vi "SimHallSensor.vi"() -> ()   [LabVIEW 2014]
doc: "Use this template to build a user interface event handler design pattern. Use this pattern for dialog boxes and other user interfaces. You also can create and execute user-defined events that the VI can handle the same way as user interface events."
uses:
  subVIs/SimHallSensor.ctl
  <vilib>/Utility/error.llb/DialogType.ctl
  <vilib>/DAQmx/create/channels.llb/DAQmx Create Channel (AO-Voltage-Basic).vi
  <vilib>/DAQmx/configure/timing.llb/DAQmx Timing (Sample Clock).vi
  <resource>/objmgr/daqmx.rc
panel:
  in  "Pulse Params":T1={"Amplitude"=5.0, "Duty Cycle"=0.1, "Shape"=enum."Square"}
  in  "Speed (RPM)":dbl(knob) scale=300.0..20000.0 scale format="%#_3p"
  in  "Engage":bool
  in  "DAQ Parameters":T2={"physical channels"="", "maximum value"=5.0, "minimum value"=-5.0, "rate"=100000.0, "buffer len"=1.0} {"buffer len" format="%0.2f"; "rate" format="%.1p"; "minimum value" format="%0.2f"; "maximum value" format="%0.2f"}
  out "Waveform Graph":waveform(dbl)(graph)
  in  "quit":bool
  # "V"
  # "V"
  # "Hz"
  # "s"
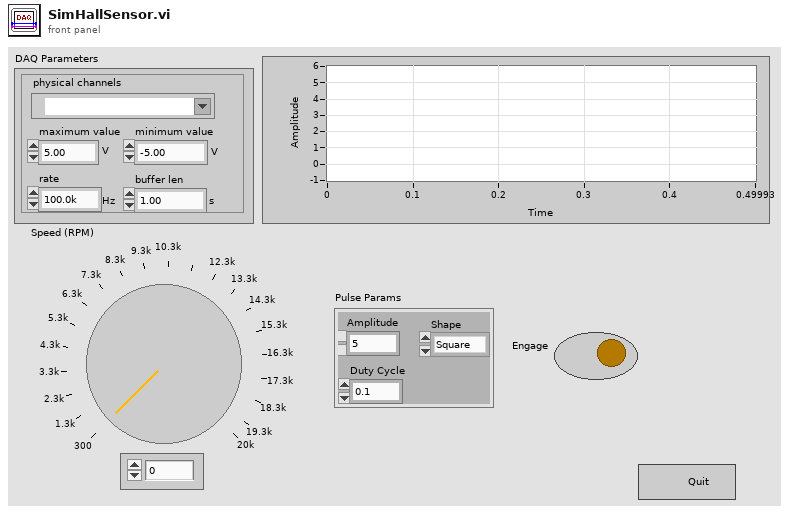
[diagram p1: front panel]
types:
  T1 = cluster{"Amplitude":dbl, "Duty Cycle":dbl, "Shape":enum16{"Square", "Cosine"}}
  T2 = cluster{"physical channels":tag, "maximum value":dbl, "minimum value":dbl, "rate":dbl, "buffer len":dbl}
  T3 = typedef "SimHallSensor.ctl" = enum16{"Init", "Idle", "CheckError", "Finalize", "ConfigDAQ", "StartDAQ", "Monitor", "StopDAQ", "ClearDAQ"}
  T4 = typedef "DialogType.ctl" = u16
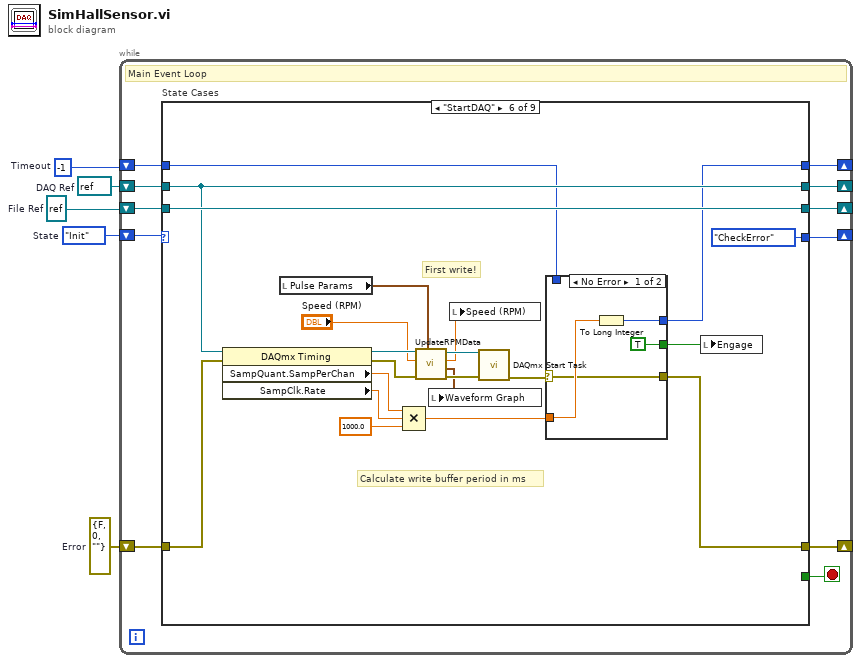
[diagram p0: block diagram]
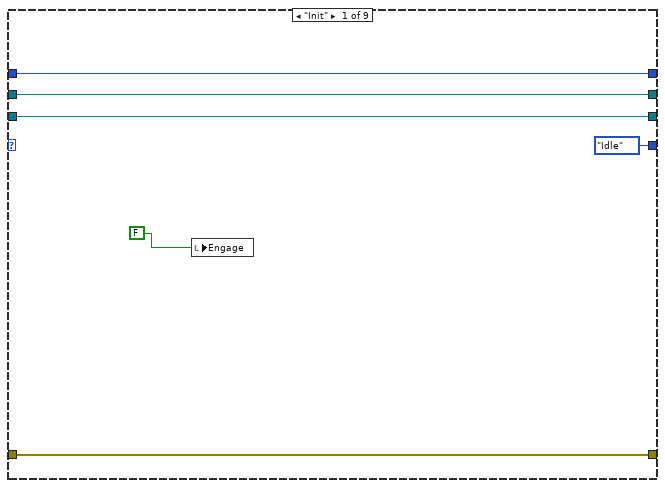
[diagram p2: hidden frame]
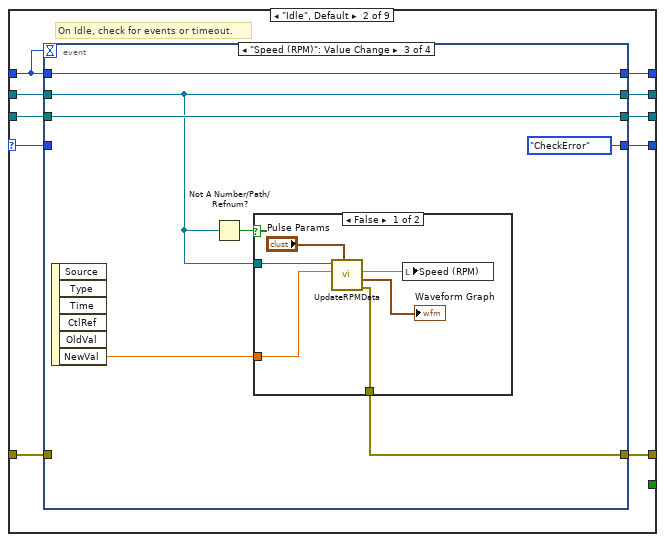
[diagram p3: hidden frame]
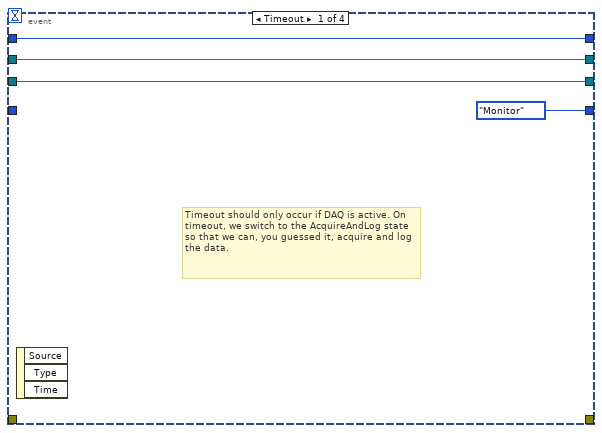
[diagram p4: hidden frame]
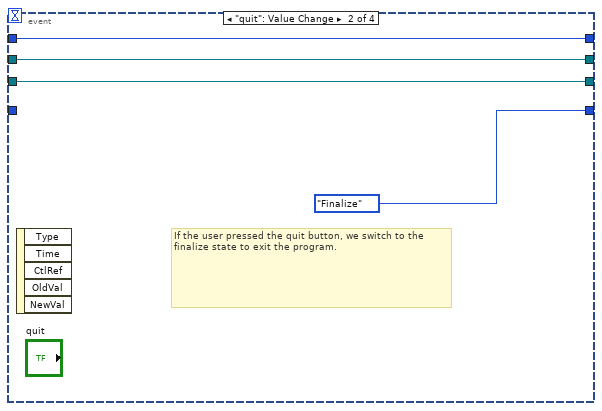
[diagram p5: hidden frame]
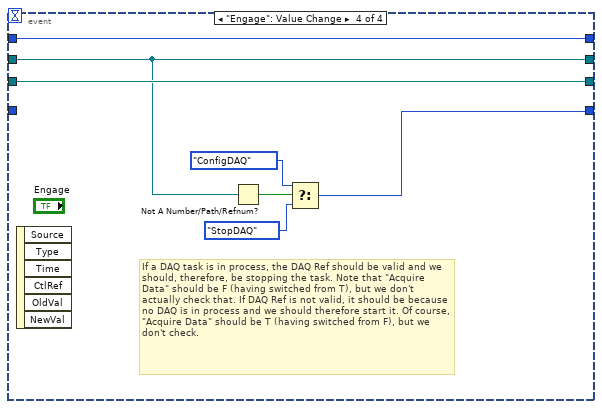
[diagram p7: hidden frame]
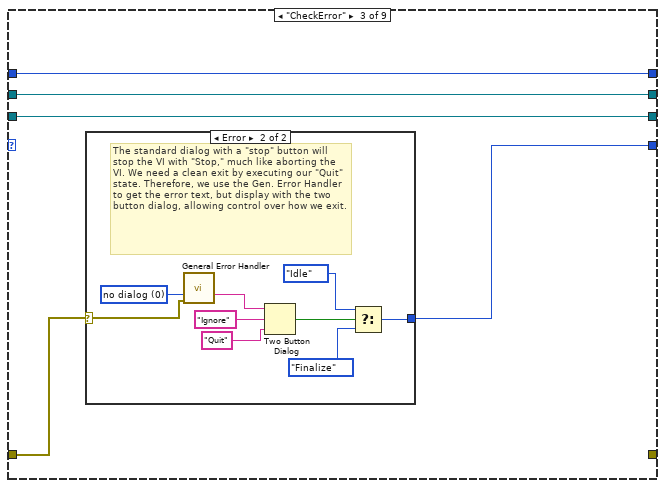
[diagram p8: hidden frame]
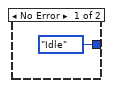
[diagram p9: hidden frame]
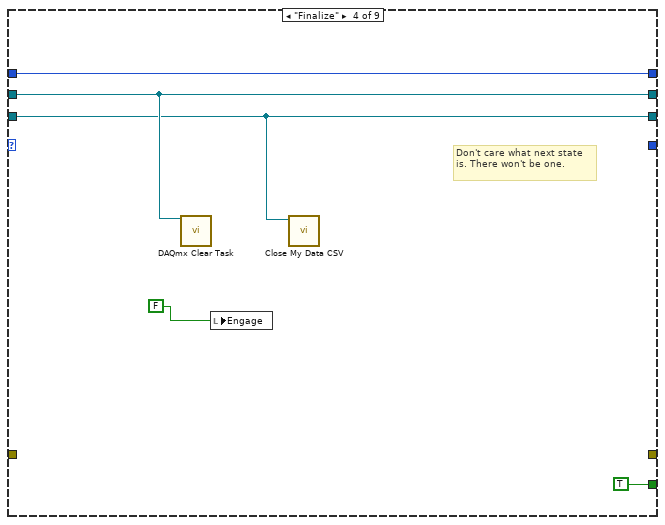
[diagram p10: hidden frame]
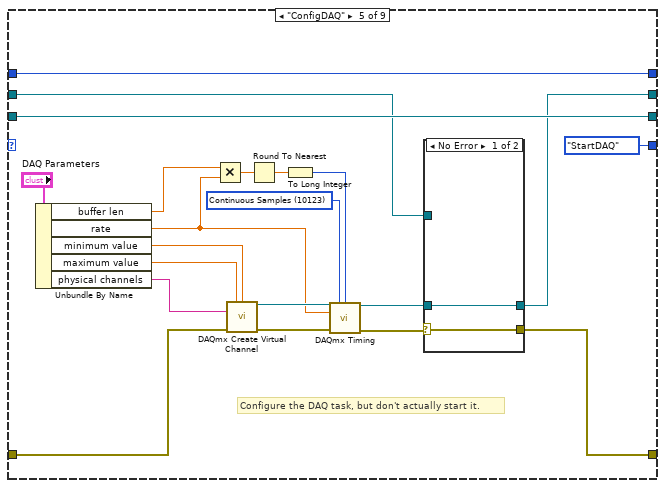
[diagram p11: hidden frame]
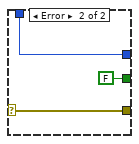
[diagram p13: hidden frame]
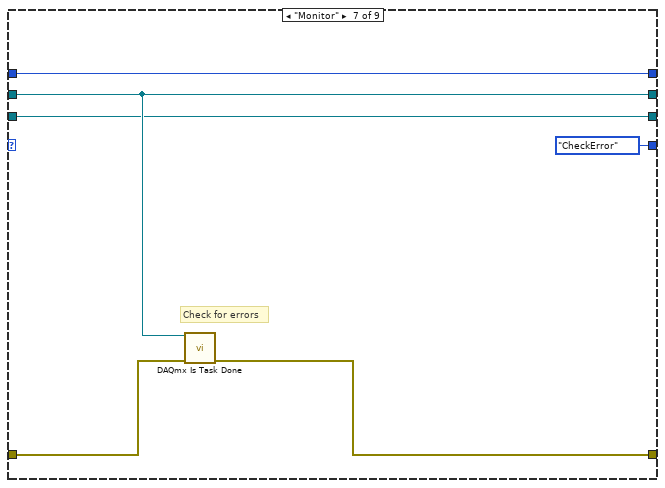
[diagram p14: hidden frame]
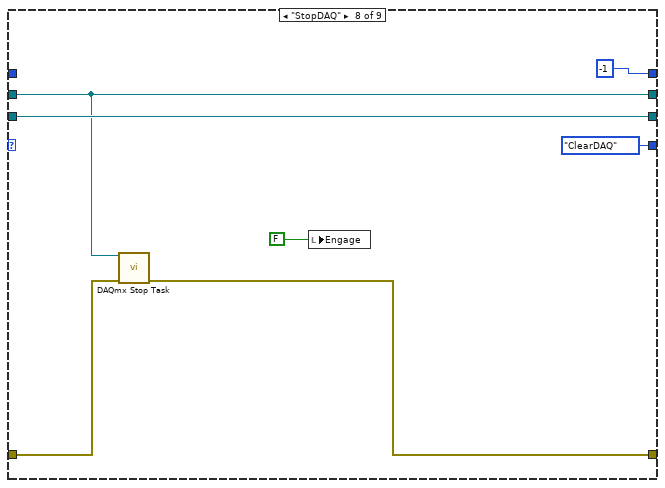
[diagram p15: hidden frame]
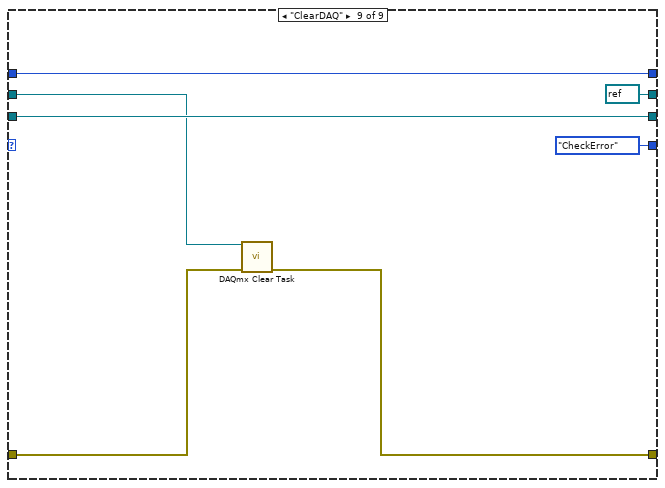
[diagram p16: hidden frame]
diagram:
  w1 = errorcluster {"status"=FALSE, "code"=0, "source"=""}  # Error
  w2 = refnum<file> refnum  # File Ref
  w3 = refnum<k21> refnum  # DAQ Ref
  w4 = SimHallSensor."Init"  # State
  w5 = -1  # Timeout
  n1 = while {
    shift-right: [w15] -> _
    shift-left: w5 -> [w16]
    shift-right: [w13] -> _
    shift-left: w4 -> [w14]
    shift-right: [w12] -> _
    shift-left: w3 -> [w11]
    shift-right: [w10] -> _
    shift-left: w2 -> [w9]
    shift-right: [w8] -> _
    shift-left: w1 -> [w7]
    stop <- w6 stop-if-true
    # "Main Event Loop"
    n2 = case "State Cases" shown="\"StartDAQ\"" w14 {
      selector: w14 -> [_ w30 _ _ _ _ _ _ _]
      tunnel: w16 -> [w22 w32 w65 w80 w89 w123 w139 _ w153]
      tunnel: [w22 w31 w65 w80 w89 w122 w139 -1 ("Timeout") w153] -> w15
      tunnel: [SimHallSensor."Idle" ("State") w29 w62 _ SimHallSensor."StartDAQ" ("State") SimHallSensor."CheckError" ("State") SimHallSensor."CheckError" ("State") SimHallSensor."ClearDAQ" ("State") SimHallSensor."CheckError" ("State")] -> w13
      tunnel: [w21 w26 w64 w78 w92 w125 w138 w141 refnum<k21> refnum ("DAQ Ref")] -> w12
      tunnel: w11 -> [w21 w25 w64 w78 w93 w125 w138 w141 w149]
      tunnel: [w20 w28 w63 w77 w101 w126 w137 w146 w151] -> w10
      tunnel: w9 -> [w20 w27 w63 w77 w101 w126 w137 w146 w151]
      tunnel: [w17 w23 _ _ w90 w121 w134 w142 w147] -> w8
      tunnel: w7 -> [w17 w24 w61 _ w83 w118 w135 w140 w148]
      tunnel: [_ _ _ TRUE _ _ _ _ _] -> w6
      frame "Init" {
        n3 = local write "Engage"(FALSE) -> ()
      }
      frame "Idle", Default {
        # "On Idle, check for events or timeout."
        # "States"
        n4 = event shown="[2] \"Speed (RPM)\": Value Change" {
          selector: _ -> [_ _ _ _]
          dyn-events: _ -> [_ _ _ _]
          timeout: w32 -> [_ _ _ _]
          tunnel: w32 -> [w36 w40 w47 w60]
          tunnel: [w36 w40 w47 w60] -> w31
          tunnel: w30 -> [_ _ _ _]
          tunnel: [SimHallSensor."Monitor" ("State") SimHallSensor."Finalize" ("State") SimHallSensor."CheckError" ("State") w54] -> w29
          tunnel: [w33 w38 w46 w59] -> w28
          tunnel: w27 -> [w33 w38 w46 w59]
          tunnel: [w35 w39 w44 w57] -> w26
          tunnel: w25 -> [w35 w39 w44 w57]
          tunnel: w24 -> [_ _ _ _]
          tunnel: [_ _ w41 _] -> w23
          event Timeout {
            # "Timeout should only occur if DAQ is active. On timeout, we switch to the AcquireAndLog state so that we can, you guessed it, acquire and log the data."
            n5 = event-data() -> ()  [unwired: 1 in, 3 out]
          }
          event "quit": Value Change {
            # "If the user pressed the quit button, we switch to the finalize state to exit the program."
            n6 = event-data() -> ()  [unwired: 1 in, 5 out]
          }
          event "Speed (RPM)": Value Change {
            n7 = event-data() -> ("NewVal"=w43:dbl)  [unwired: 1 in, 5 out]
            n8 = Not A Number/Path/Refnum?(number/path/refnum=w44) -> (NaN/Path/Refnum?=w45:bool)
            n9 = case shown="False" w45 {
              tunnel: w44 -> [w53 _]
              tunnel: w43 -> [w50 _]
              tunnel: [w49 _] -> w41
              frame False {
                n10 = call "UpdateRPMData.vi"("Pulse Params"="Pulse Params", "RPM"=w50, "Refnum in"=w53) -> ("error out"=w49:errorcluster, "Waveform"=→"Waveform Graph":waveform(dbl), "RPM out"=w52:dbl)  [unwired: 3 in, 1 out]
                n11 = local write "Speed (RPM)"(w52) -> ()
              }
              frame True {
              }
            }
          }
          event "Engage": Value Change {
            # "If a DAQ task is in process, the DAQ Ref should be valid and we should, therefore, be stopping the task. Note that \"Acquire Data\" should be F (having switched from T), but we don't actually check that. If DAQ Ref is not valid, it should be because no DAQ is in process and we should therefore start it. Of course, \"Acquire Data\" should be T (having switched from F), but we don't check."
            n12 = event-data() -> ()  [unwired: 1 in, 6 out]
            n13 = Not A Number/Path/Refnum?(number/path/refnum=w57) -> (NaN/Path/Refnum?=w58:bool)
            n14 = Select(t=SimHallSensor."ConfigDAQ" ("State"), s=w58, f=SimHallSensor."StopDAQ" ("State")) -> (s? t:f=w54:T3)
          }
        }
      }
      frame "CheckError" {
        n15 = case shown="Error" w61 {
          selector: w61 -> [_ w67]
          tunnel: [SimHallSensor."Idle" ("State") w68] -> w62
          frame No Error {
          }
          frame Error {
            w75 = T4 0 items=["no dialog", "OK message", "continue or stop message", "OK message + warnings", "continue/stop + warnings"] ("type of dialog (OK msg:1)")
            # "The standard dialog with a \"stop\" button will stop the VI with \"Stop,\" much like aborting the VI. We need a clean exit by executing our \"Quit\" state. Therefore, we use the Gen. Error Handler to get the error text, but display with the two button dialog, allowing control over how we exit."
            n16 = call <vilib>:"General Error Handler.vi"("type of dialog (OK msg:1)"=w75, "error in (no error)"=w67) -> ("message"=w74:string)  [unwired: 9 in, 4 out]
            n17 = Two Button Dialog(message=w74, 1:"Quit" ("F button name (\"Cancel\")"), 2:"Ignore" ("T button name (\"OK\")")) -> (T button?=w71:bool)
            n18 = Select(t=SimHallSensor."Idle" ("State"), s=w71, f=SimHallSensor."Finalize" ("State")) -> (s? t:f=w68:T3)
          }
        }
      }
      frame "Finalize" {
        # "Don't care what next state is. There won't be one."
        n19 = call <vilib>:"DAQmx Clear Task.vi"("task in"=w78) -> ()  [unwired: 14 in, 1 out]
        n20 = local write "Engage"(FALSE) -> ()
        n21 = call "Close My Data CSV.vi"("file refnum"=w77) -> ()  [unwired: 10 in, 1 out]
      }
      frame "ConfigDAQ" {
        w98 = 10123 items=["Finite Samples"=10178, "Continuous Samples"=10123, "Hardware Timed Single Point"=12522] ("sample mode")
        # "Configure the DAQ task, but don't actually start it."
        n22 = Unbundle By Name("DAQ Parameters") -> ("buffer len"=w87:dbl, "rate"=w82:dbl, "minimum value"=w86:dbl, "maximum value"=w85:dbl, "physical channels"=w84:tag)
        n23 = Multiply(x=w87, y=w82) -> (x*y=w97:dbl)
        n24 = call-poly <vilib>:"DAQmx Create Virtual Channel.vi"("maximum value"=w85, "minimum value"=w86, "physical channels"=w84, "error in"=w83) -> ("task out"=w100:refnum<k21>, "error out"=w99:errorcluster)  [unwired: 10 in]
        n25 = Round To Nearest(number=w97) -> (nearest integer value=w96:dbl)
        n26 = To Long Integer(number=w96) -> (32bit integer=w95:i32)
        n27 = call-poly <vilib>:"DAQmx Timing.vi"("task/channels in"=w100, "sample mode"=w98, "samples per channel"=w95, "rate"=w82, "error in"=w99) -> ("task out"=w91:refnum<k21>, "error out"=w94:errorcluster)  [unwired: 9 in]
        n28 = case shown="No Error" w94 {
          selector: w94 -> [w102 w105]
          tunnel: w93 -> [_ w104]
          tunnel: [w103 w104] -> w92
          tunnel: w91 -> [w103 _]
          tunnel: [w102 w105] -> w90
          frame No Error {
          }
          frame Error {
          }
        }
      }
      frame "StartDAQ" {
        # "First write!"
        # "Calculate write buffer period in ms"
        n29 = property class="DAQmx Timing"(reference=w125, error in=w118) -> (reference out=w113:refnum<k21>, error out=w111:errorcluster, "SampQuant.SampPerChan"=w117:dbl, "SampClk.Rate"=w116:dbl)
        n30 = local read "Pulse Params"() -> (w106:T1)
        n31 = Compound Arithmetic op=MULTIPLY(w117, w116, 1000.0 ("value")) -> (w114:dbl)
        n32 = call "UpdateRPMData.vi"("Pulse Params"=w106, "error in (no error)"=w111, "RPM"="Speed (RPM)", "Refnum in"=w113) -> ("error out"=w110:errorcluster, "Waveform"=w107:waveform(dbl), "RPM out"=w108:dbl, "Refnum out"=w112:refnum<k21>)  [unwired: 2 in]
        n33 = local write "Waveform Graph"(w107) -> ()
        n34 = local write "Speed (RPM)"(w108) -> ()
        n35 = call <vilib>:"DAQmx Start Task.vi"("task/channels in"=w112, "error in"=w110) -> ("error out"=w124:errorcluster)  [unwired: 12 in, 1 out]
        n36 = case shown="No Error" w124 {
          selector: w124 -> [w128 w132]
          tunnel: w114 -> [w130 _]
          tunnel: w123 -> [_ w133]
          tunnel: [w129 w133] -> w122
          tunnel: [w128 w132] -> w121
          tunnel: [TRUE FALSE] -> w119
          frame No Error {
            n37 = To Long Integer(number=w130) -> (32bit integer=w129:i32)
          }
          frame Error {
          }
        }
        n38 = local write "Engage"(w119) -> ()
      }
      frame "Monitor" {
        # "Check for errors"
        n39 = call <vilib>:"DAQmx Is Task Done.vi"("task/channels in"=w138, "error in"=w135) -> ("error out"=w134:errorcluster)  [unwired: 11 in, 2 out]
      }
      frame "StopDAQ" {
        n40 = call <vilib>:"DAQmx Stop Task.vi"("task/channels in"=w141, "error in"=w140) -> ("error out"=w142:errorcluster)  [unwired: 12 in, 1 out]
        n41 = local write "Engage"(FALSE ("Acquire Data")) -> ()
      }
      frame "ClearDAQ" {
        n42 = call <vilib>:"DAQmx Clear Task.vi"("task in"=w149, "error in"=w148) -> ("error out"=w147:errorcluster)  [unwired: 13 in]
      }
    }
  }
